vi "APDM Sync Sensors.vi"(3 "error in (no error)":errorcluster, 5 "APDM Context":T1={"APDM Context ID"=0, "Gyro Mode"="", "Log Data"=FALSE, "Log File"=refnum, "Gyro Record Log"=refnum, "Gyro CMD Log"=refnum, "L Opal SN"=0, "R Opal SN"=0, "Access Point ID"=0, "Left Gyro Sim Data"=path "C:/Users/jfalesi/Desktop/CP FES Walking Code/Original/Ahad Vi/CP Code/Offline data/TD_7_Raw_R.txt", "Right Gyro Sim Data"=path "C:/Users/jfalesi/Desktop/CP FES Walking Code/Original/Ahad Vi/CP Code/Offline data/TD_7_Raw_R.txt", "Sampling Rate"=0.0, "Gyro Sim Time Array"=[], "Missed Gyro Count"=0.0}) -> (0 "error out":errorcluster, 2 "APDM Context":T1={"APDM Context ID"=0, "Gyro Mode"="", "Log Data"=FALSE, "Log File"=refnum, "Gyro Record Log"=refnum, "Gyro CMD Log"=refnum, "L Opal SN"=0, "R Opal SN"=0, "Access Point ID"=0, "Left Gyro Sim Data"=path "C:/Users/jfalesi/Desktop/CP FES Walking Code/Original/Ahad Vi/CP Code/Offline data/TD_7_Raw_R.txt", "Right Gyro Sim Data"=path "C:/Users/jfalesi/Desktop/CP FES Walking Code/Original/Ahad Vi/CP Code/Offline data/TD_7_Raw_R.txt", "Sampling Rate"=0.0, "Gyro Sim Time Array"=[], "Missed Gyro Count"=0.0})   [LabVIEW 2019]
uses:
  Controls/APDM Context Cluster.ctl
  Lee Lab/CP FES Walking 2018/Code/Working/LabVIEW/apdm.dll
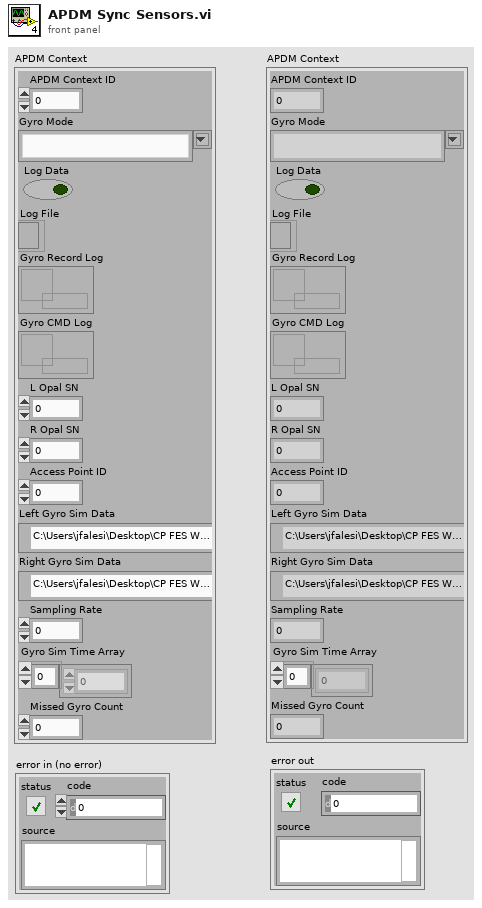
[diagram p1: front panel]
types:
  T1 = typedef "APDM Context Cluster.ctl" = cluster{"APDM Context ID":u32, "Gyro Mode":string, "Log Data":bool, "Log File":refnum<file>, "Gyro Record Log":refnum<queue>, "Gyro CMD Log":refnum<queue>, "L Opal SN":u32, "R Opal SN":u32, "Access Point ID":u32, "Left Gyro Sim Data":path, "Right Gyro Sim Data":path, "Sampling Rate":dbl, "Gyro Sim Time Array":dbl[], "Missed Gyro Count":dbl}
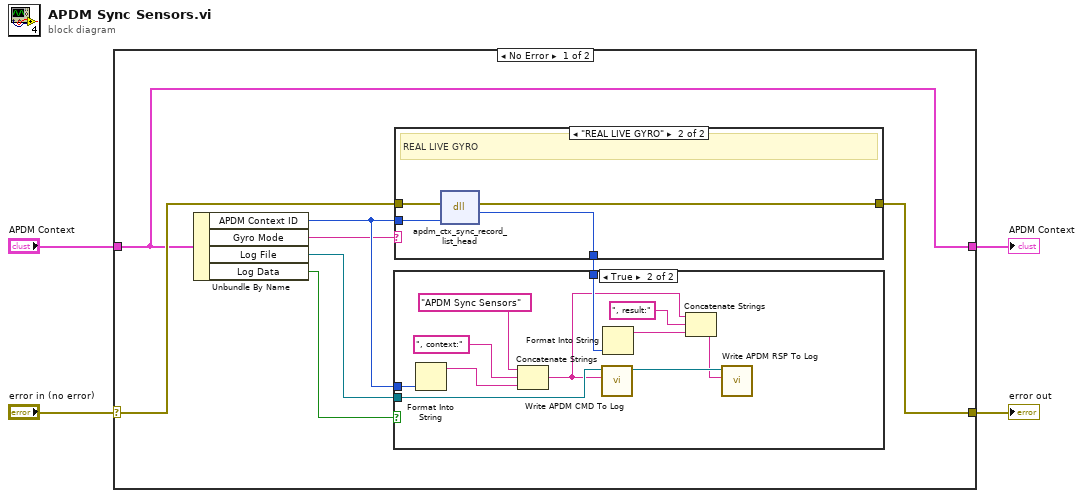
[diagram p0: block diagram]
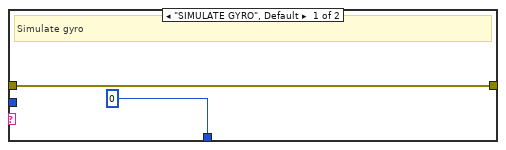
[diagram p3: hidden frame]
diagram:
  n1 = case shown="No Error" "error in (no error)" {
    selector: "error in (no error)" -> [w7 w31]
    tunnel: [w6 w31] -> w3
    tunnel: "APDM Context" -> [w5 w30]
    tunnel: [w5 w30] -> w1
    frame No Error {
      n2 = Unbundle By Name(w5) -> ("APDM Context ID"=w11:u32, "Gyro Mode"=w8:string, "Log File"=w9:refnum<file>, "Log Data"=w10:bool)
      n3 = case shown="\"REAL LIVE GYRO\"" w8 {
        tunnel: w11 -> [_ w29]
        tunnel: w7 -> [w25 w28]
        tunnel: [w25 w27] -> w6
        tunnel: [0 w26] -> w12
        frame "SIMULATE GYRO", Default {
          # "Simulate gyro"
        }
        frame "REAL LIVE GYRO" {
          # "REAL LIVE GYRO"
          n4 = dll-call lib="C:/Users/jfalesi/Dropbox/Lee Lab/CP FES Walking 2018/Code/Working/LabVIEW/apdm.dll" fn="apdm_ctx_sync_record_list_head"(error in=w28, "context"=w29) -> (error out=w27:errorcluster, "return type"=w26:i32)  [unwired: 3 in, 1 out]
        }
      }
      n5 = case shown="True" w10 {
        tunnel: w11 -> [_ w20]
        tunnel: w12 -> [_ w15]
        tunnel: w9 -> [_ w14]
        frame False {
        }
        frame True {
          n6 = Format Into String(w20) -> (resulting string=w21:string)  [unwired: 3 in, 1 out]
          n7 = Concatenate Strings("APDM Sync Sensors" ("Log Item"), ", context:" ("string"), w21) -> (w13:string)
          n8 = call "Write APDM CMD To Log.vi"("Log Item"=w13, "Byte Stream File in"=w14) -> ("Byte Stream File out"=w23:refnum<file>)  [unwired: 8 in, 1 out]
          n9 = Format Into String(w15) -> (resulting string=w19:string)  [unwired: 3 in, 1 out]
          n10 = Concatenate Strings(w13, ", result:" ("string"), w19) -> (w17:string)
          n11 = call "Write APDM RSP To Log.vi"("Log Item"=w17, "Byte Stream File in"=w23) -> ()  [unwired: 9 in, 1 out]
        }
      }
    }
    frame Error {
    }
  }
  "error out" <- w3
  "APDM Context" <- w1
